vi "Out_S1F3.vi"(8 "error in (no error)":errorcluster, 10 "Status Variable ID(SVID)":u32[](array[numeric]), 11 "S1 Message Class in":refnum<class "S1 Message Class.lvclass">) -> (0 "error out":errorcluster, 3 "S1 Message Class out":refnum<class "S1 Message Class.lvclass">)   [LabVIEW 2020, in "SECS Communication.lvlib" / "S1 Message Class.lvclass"]
uses:
  S1 Message Class.lvclass
  D:/Dropbox/SECS/LabVIEW Code/Com/SECS Communication/SECS-II Class/SECS-II Class.lvclass
  SECS-II Class/Data Message_List.vi
  SECS-II Class/Data Message_U4.vi
  S1 Message Class.lvclass/S1 Message Class.ctl
  SECS-II Class/SECS-II Class.lvclass
  D:/Dropbox/SECS/LabVIEW Code/Com/SECS Communication/S1 Message Class/S1 Message Class.lvclass
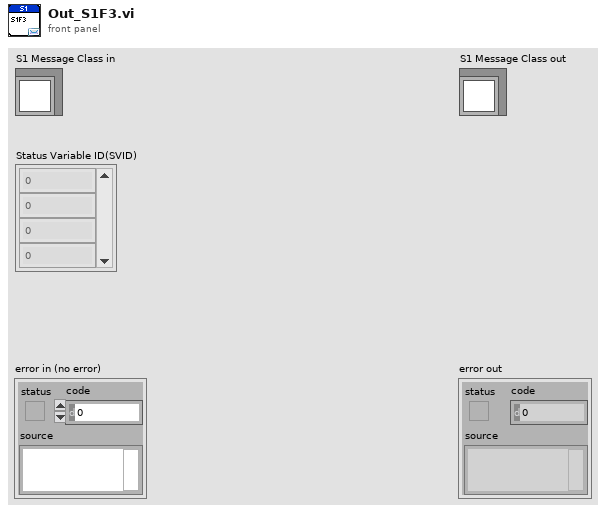
[diagram p1: front panel]
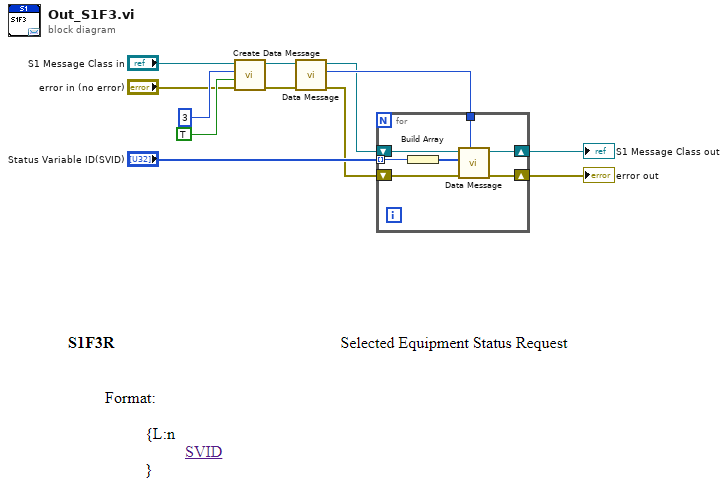
[diagram p0: block diagram]
diagram:
  n1 = call "Create Data Message.vi"("error in (no error)"="error in (no error)", "W-Bit"=TRUE, "Function"=u8 3, "SECS-II Class in"="S1 Message Class in") -> ("error out"=w5:errorcluster, "SECS-II Class out"=w6:refnum<class "S1 Message Class.lvclass">)  [unwired: 6 in]
  n2 = call-poly "Data Message.vi"("error in"=w5, "SECS-II Class in"=w6) -> ("error out"=w3:errorcluster, "Index"=w7:i32, "SECS-II Class out"=w2:refnum<class "S1 Message Class.lvclass">)  [unwired: 7 in]
  n3 = for {
    tunnel: w7 -> [w18]
    tunnel: "Status Variable ID(SVID)" -> [w14] mode=indexing
    shift-right: [w19] -> w8
    shift-left: w3 -> [w17]
    shift-right: [w15] -> w1
    shift-left: w2 -> [w16]
    n4 = Build Array(w14) -> (w13:u32[])
    n5 = call-poly "Data Message.vi"("Parent Index"=w18, "error in"=w17, "Data"=w13, "SECS-II Class in"=w16) -> ("error out"=w19:errorcluster, "SECS-II Class out"=w15:refnum<class "S1 Message Class.lvclass">)  [unwired: 6 in]
  }
  "error out" <- w8
  "S1 Message Class out" <- w1
